vi "Register Relay Appender.vi"(4 "queueBound":i32=-1, 6 "filter":T2={"mode"=enum."Mirror", "levelMin"=enum."INFO", "levelMax"=enum."INFO", "tagPrefix"=""}, 8 "error in (no error)":errorcluster, 9 "threshold":T1=enum."ALL", 10 "id in":string, 11 "Logger in":refnum<class "Logger.lvclass">) -> (0 "error out":errorcluster, 1 "relayQueue":refnum<queue>, 2 "id out":string, 3 "Logger out":refnum<class "Logger.lvclass">)   [LabVIEW 2026, in "Tests.lvlib"]
doc: "Test-support Arrange step. Given a live logger and a unique id, builds a queue-mode relay appender, registers it (which blocks on WaitForSnapshot, so it's live on return), and hands back the queue refnum the test drains to observe delivery."
uses:
  Tests.lvlib
  src/Public/Logger.lvclass/Logger.lvclass
  src/TypeDefs/Statement.ctl
  src/TypeDefs/Severity.ctl
  src/TypeDefs/Filter.ctl
  src/TypeDefs/FilterMode.ctl
  src/TypeDefs/AppenderConfig.ctl
  src/TypeDefs/DropPolicy.ctl
  src/TypeDefs/RelayMode.ctl
  src/Core/Appenders/RelayAppender.lvclass/RelayAppender.lvclass
  C:/Users/dallis/OneDrive - Velico Medical/Documents/Personal/LabVIEW Coding Projects/Lumberjack/src/Core/Appenders/Appender.lvclass/Appender.lvclass
  C:/Program Files (x86)/National Instruments/LabVIEW 2026/vi.lib/ActorFramework/Actor/Actor.lvclass
  C:/Users/dallis/OneDrive - Velico Medical/Documents/Personal/LabVIEW Coding Projects/Lumberjack/src/Core/Appenders/RelayAppender.lvclass/RelayAppender.lvclass
  src/Lumberjack.lvlib
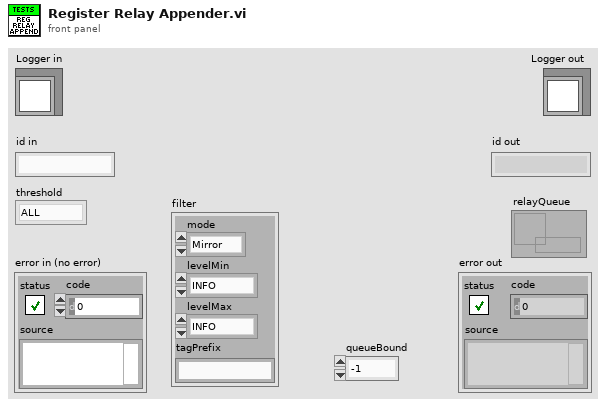
[diagram p1: front panel]
types:
  T1 = typedef "Lumberjack.lvlib/Severity.ctl" = enum16{"OFF", "FATAL", "ERROR", "WARN", "INFO", "DEBUG", "TRACE", "ALL"}
  T2 = typedef "Lumberjack.lvlib/Filter.ctl" = cluster{"mode":T3, "levelMin":T1, "levelMax":T1, "tagPrefix":string}
  T3 = typedef "Lumberjack.lvlib/FilterMode.ctl" = enum16{"Mirror", "Routed"}
  T4 = typedef "Lumberjack.lvlib/RelayMode.ctl" = enum16{"Message", "Queue"}
  T5 = typedef "Lumberjack.lvlib/AppenderConfig.ctl" = cluster{"id":string, "threshold":T1, "filter":T2, "queueBound":i32, "dropPolicy":T6, "useUTC":bool}
  T6 = typedef "Lumberjack.lvlib/DropPolicy.ctl" = enum16{"DropOldest", "DropNewest", "LevelAware"}
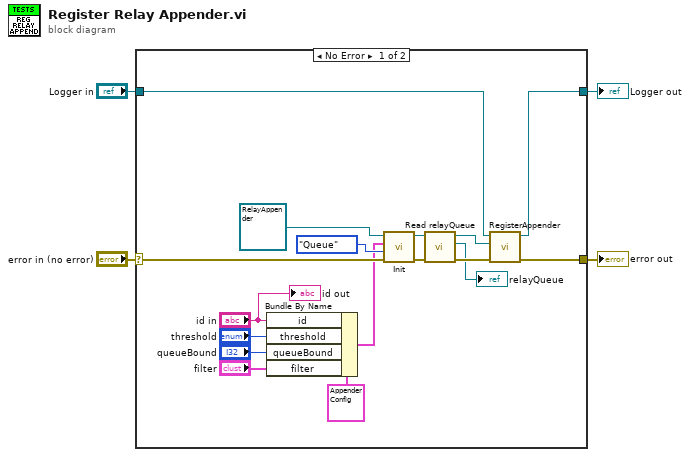
[diagram p0: block diagram]
diagram:
  n1 = case shown="No Error" "error in (no error)" {
    selector: "error in (no error)" -> [w12 w23]
    tunnel: [w5 w23] -> w3
    tunnel: [w7 w22] -> w1
    tunnel: "Logger in" -> [w8 w22]
    frame No Error {
      n2 = Bundle By Name(cluster=T5 {"id"="", "threshold"=enum."INFO", "filter"={"mode"=enum."Mirror", "levelMin"=enum."INFO", "levelMax"=enum."INFO", "tagPrefix"=""}, "queueBound"=0, "dropPolicy"=enum."DropOldest", "useUTC"=FALSE} ("AppenderConfig"), "id"="id in", "threshold"="threshold", "queueBound"="queueBound", "filter"="filter") -> (w11:T5)
      n3 = call "Init.vi"("error in (no error)"=w12, "mode"=RelayMode."Queue", "common"=w11, "RelayAppender in"=refnum<class "RelayAppender.lvclass"> refnum) -> ("error out"=w18:errorcluster, "RelayAppender out"=w17:refnum<class "RelayAppender.lvclass">)  [unwired: 6 in]
      n4 = call "Read relayQueue.vi"("error in (no error)"=w18, "RelayAppender in"=w17) -> ("error out"=w16:errorcluster, "relayQueue"=→"relayQueue":refnum<queue>, "RelayAppender out"=w15:refnum<class "RelayAppender.lvclass">)  [unwired: 7 in]
      n5 = call "RegisterAppender.vi"("error in (no error)"=w16, "Lumberjack.lvlib:Appender.lvclass"=w15, "Logger in"=w8) -> ("error out"=w5:errorcluster, "Logger out"=w7:refnum<class "Logger.lvclass">)  [unwired: 7 in]
      "id out" <- "id in"
    }
    frame Error {
    }
  }
  "error out" <- w3
  "Logger out" <- w1
